vi "Autolocate Fiducials.vi"(6 "FD Index":i32, 8 "error in":errorcluster, 9 "Past Fiducials":dbl[](array[numeric]), 10 "Component":T1, 11 "Gantry In":refnum<k24>) -> (0 "error out":errorcluster, 1 "Wrong Orientation?":bool, 2 "Component Out":T1, 3 "Gantry Out":refnum<k24>)   [LabVIEW 2021, in "Component Tray.lvclass"]
uses:
  Component Tray.lvclass
  C:/Program Files (x86)/Aerotech/A3200/LabVIEW/2010/Bin/Aerotech.A3200.dll
  Program Files (x86)/Aerotech/A3200/LabVIEW/2010/Bin/Aerotech.A3200.dll
  Find Component.ctl
  Controller/Camera/Machine Vision.ctl
  Controller/Motion/A3200/A3200.lvclass
  Controller/Motion/Motion.lvclass
  Controller/Camera/Camera.lvclass
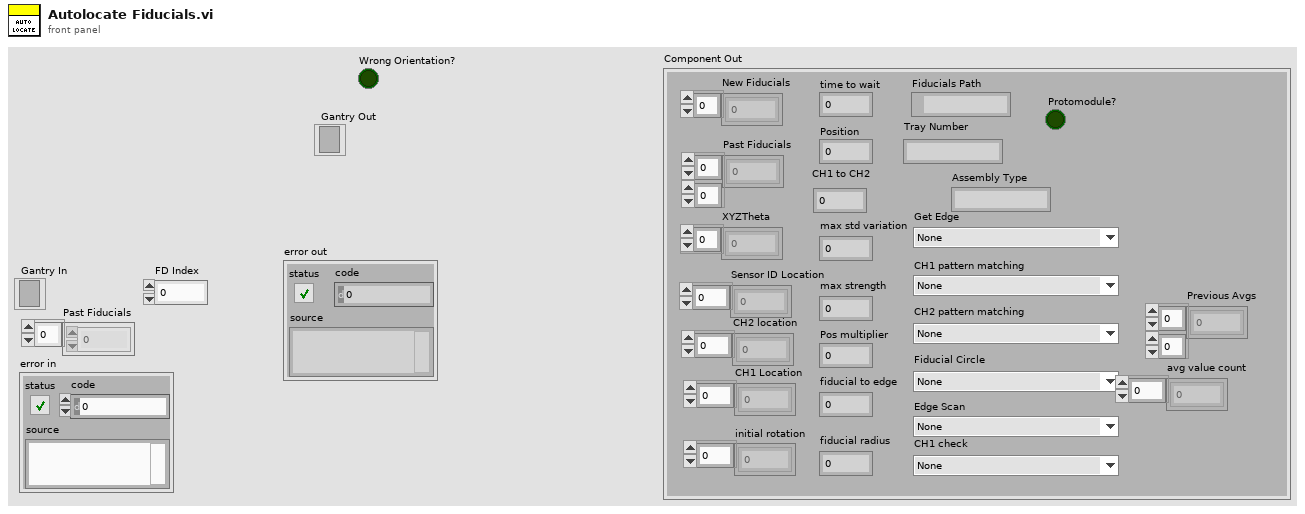
[diagram p1: front panel]
types:
  T1 = typedef "Component Tray.lvclass/Find Component.ctl" = cluster{"New Fiducials":dbl[], "Past Fiducials":dbl[][], "XYZTheta":dbl[], "Fiducials Path":path, "Position":i32, "CH1 Location":dbl[], "Sensor ID Location":dbl[], "initial rotation":dbl[], "CH2 location":dbl[], "max std variation":dbl, "max strength":dbl, "CH2 pattern matching":T2, "Fiducial Circle":T2, "Get Edge":T2, "Pos multiplier":dbl, "time to wait":u32, "fiducial to edge":dbl, "Protomodule?":bool, "Assembly Type":string, "CH1 to CH2":dbl, "Tray Number":string, "fiducial radius":dbl, "4 fiducials?":bool, "CH1 check":T2, "Edge Scan":T2, "CH1 pattern matching":T2, "Sensor Thickness":dbl, "Previous Avgs":dbl[][], "avg value count":dbl[]}
  T2 = typedef "Camera.lvclass/Machine Vision.ctl" = enum16{"None", "Assembly Tray Circle", "Assembly Tray Fiducial", "Partial Hexaboard", "sensor edge init", "HB edge init", "sensor edge pos1", "sensor edge pos2", "HB edge pos1", "HB edge pos2", "Sensor CH1-2", "HB CH1", "HB CH2", "V3 Sensor Circle", "Hexaboard Circle", "sensor CH1 check", "HB CH1 check ", "sensor ID"}
  T3 = enum16{"None", "Assembly Tray Circle", "Assembly Tray Fiducial", "Partial Hexaboard", "sensor edge init", "HB edge init", "sensor edge pos1", "sensor edge pos2", "HB edge pos1", "HB edge pos2", "Sensor CH1-2", "HB CH1", "HB CH2", "V3 Sensor Circle", "Hexaboard Circle", "sensor CH1 check", "HB CH1 check "}
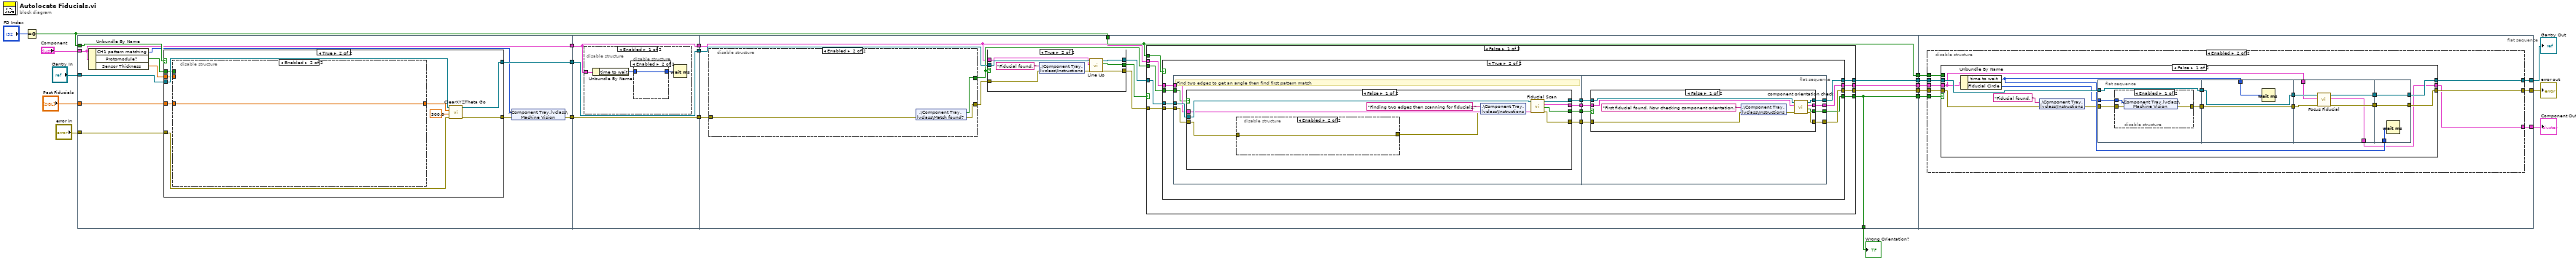
[diagram p0: block diagram]
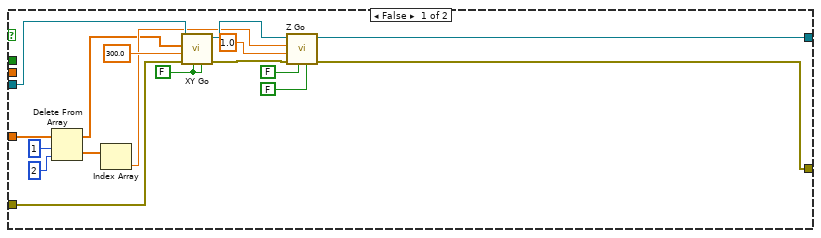
[diagram p2: hidden frame]
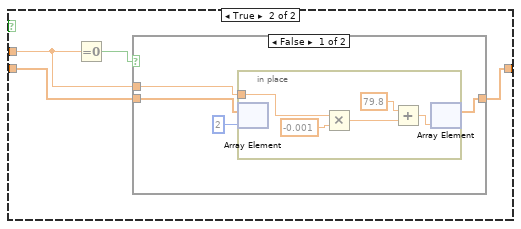
[diagram p4: hidden frame]
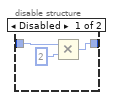
[diagram p6: hidden frame]
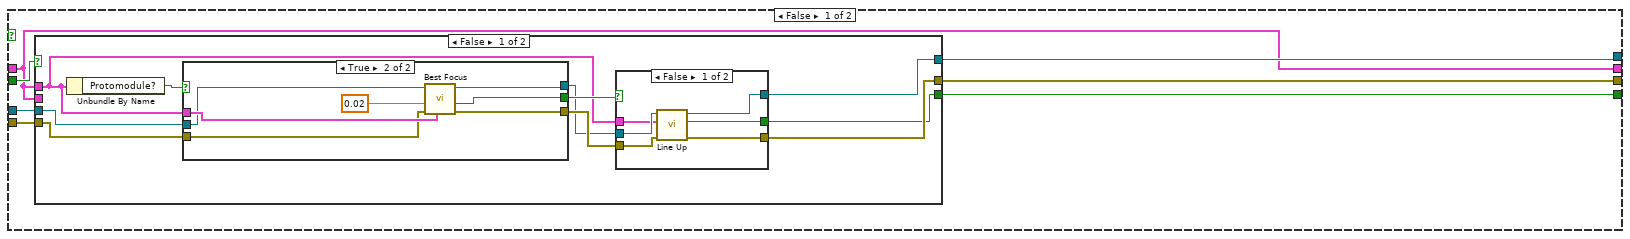
[diagram p8: hidden frame]
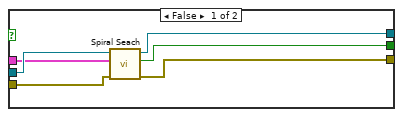
[diagram p9: hidden frame]
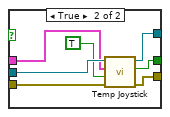
[diagram p10: hidden frame]
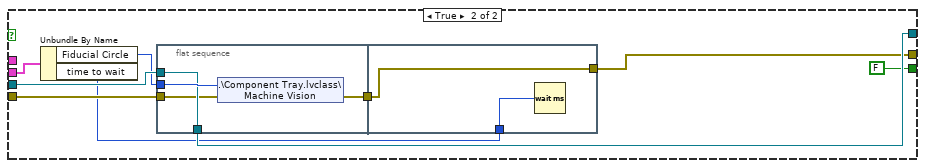
[diagram p11: hidden frame]
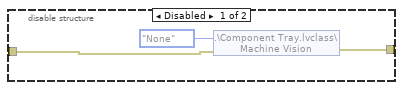
[diagram p12: hidden frame]
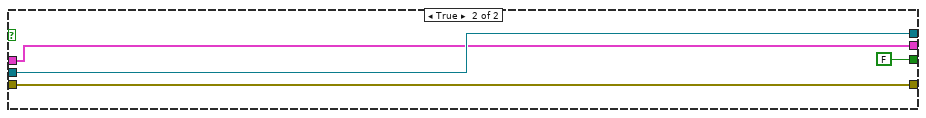
[diagram p13: hidden frame]
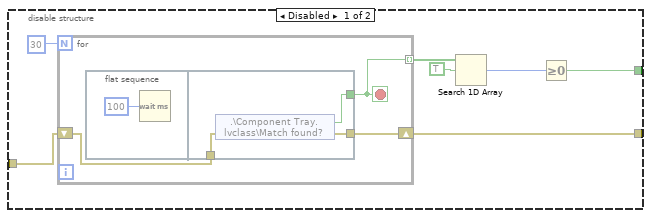
[diagram p16: hidden frame]
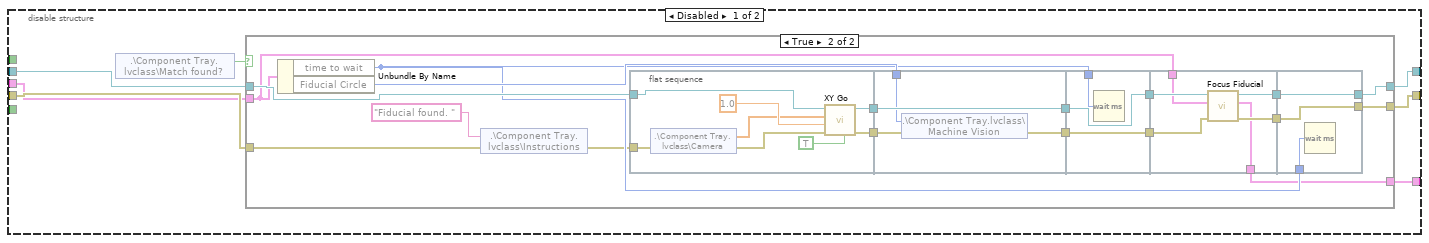
[diagram p18: hidden frame]
diagram:
  n1 = Equal To 0?(x="FD Index") -> (x = 0?=w17:bool)
  n2 = flat-sequence {
    tunnel: w17 -> [w32]
    tunnel: "Gantry In" -> [w31]
    tunnel: "Past Fiducials" -> [w30]
    tunnel: "error in" -> [w24]
    tunnel: [w29] -> w10
    tunnel: "Component" -> [w28]
    tunnel: [w28] -> w11
    tunnel: [w22] -> w9
    tunnel: w11 -> [w81]
    tunnel: [w81] -> w6
    tunnel: [w80] -> w5
    tunnel: w10 -> [w79]
    tunnel: [w79] -> w4
    tunnel: w9 -> [w80]
    tunnel: w17 -> [w97]
    tunnel: [w101] -> w16
    tunnel: [w99] -> w15
    tunnel: [w100] -> w13
    tunnel: [w98] -> w12
    tunnel: [w98] -> w8
    tunnel: [w97] -> w7
    tunnel: w4 -> [w93]
    tunnel: w5 -> [w96]
    tunnel: w6 -> [w90]
    tunnel: [w267] -> w1
    tunnel: [w266] -> w3
    tunnel: w16 -> [w265]
    tunnel: w15 -> [w263]
    tunnel: [w262] -> w2
    tunnel: w13 -> [w264]
    tunnel: w8 -> [w261]
    tunnel: w7 -> [w260]
    frame #0 {
      n3 = Unbundle By Name(w28) -> ("CH1 pattern matching"=w27:T2, "Protomodule?"=w26:bool, "Sensor Thickness"=w25:dbl)
      n4 = case shown="True" w32 {
        tunnel: w30 -> [w45 w54]
        tunnel: w31 -> [w49 w58]
        tunnel: [w43 w57] -> w29
        tunnel: w24 -> [w47 w56]
        tunnel: w26 -> [_ w50]
        tunnel: [w42 w55] -> w23
        tunnel: w25 -> [_ w53]
        frame False {
          w48 = FALSE ("Increment?")
          n5 = Delete From Array(array=w45, length=1, index=2) -> (deleted portion=w35:dbl[], array with subset deleted=w33:dbl[])
          n6 = Index Array(array=w35) -> (element=w34:dbl)  [unwired: 1 in]
          n7 = call "XY Go.vi"("Increment?"=w48, "return immediately"=w48, "error in (no error)"=w47, "Speed"=300.0, "XY In"=w33, "Gantry In"=w49) -> ("error out"=w41:errorcluster, "Gantry Out"=w44:refnum<k24>)  [unwired: 3 in, 1 out]
          n8 = call "Z Go.vi"("Increment"=FALSE, "Return Immediately"=FALSE, "error in (no error)"=w41, "Speed In"=1.0, "Position In"=w34, "Gantry In"=w44) -> ("error out"=w42:errorcluster, "Gantry Out"=w43:refnum<k24>)  [unwired: 2 in, 2 out]
        }
        frame True {
          n9 = disable-structure shown="Enabled" {
            disable-tunnel: w54 -> [w62 w78]
            disable-tunnel: w53 -> [w61 _]
            disable-tunnel: [w60 w78] -> w52
            disable-tunnel: w50 -> [w59 _]
            frame Disabled {
              n10 = case shown="False" w59 {
                tunnel: w62 -> [w63 w66]
                tunnel: w61 -> [_ w65]
                tunnel: [w63 w64] -> w60
                frame False {
                }
                frame True {
                  n11 = Equal To 0?(x=w65) -> (x = 0?=w67:bool)
                  n12 = case shown="False" w67 {
                    tunnel: w66 -> [w71 w77]
                    tunnel: w65 -> [w70 _]
                    tunnel: [w69 w77] -> w64
                    frame False {
                      n13 = in-place {
                        in-place-border: w70 -> [w75]
                        n14 = in-place-array #1(w71, 2) -> ()  [unwired: 1 out]
                        n15 = Multiply(x=w75, y=-0.001) -> (x*y=w73:dbl)
                        n16 = Add(x=79.8, y=w73) -> (x+y=w72:dbl)
                        n17 = in-place-array #1(w72) -> (w69:dbl[])  [unwired: 1 out]
                      }
                    }
                    frame True {
                    }
                  }
                }
              }
            }
            frame Enabled {
            }
          }
          n18 = call "ClearXYZTheta Go.vi"("error in (no error)"=w56, "Speed"=300.0, "XYZTheta In"=w52, "Gantry In"=w58) -> ("error out"=w55:errorcluster, "Gantry Out"=w57:refnum<k24>)  [unwired: 5 in, 1 out]
        }
      }
      n19 = shared-variable ".\\Component Tray.lvclass\\Machine Vision"(w27, error in=w23) -> (error out=w22:errorcluster)
    }
    frame #1 {
      n20 = disable-structure shown="Enabled" {
        disable-tunnel: w81 -> [w84 _]
        frame Enabled {
          n21 = Unbundle By Name(w84) -> ("time to wait"=w83:u32)
          n22 = disable-structure shown="Enabled" {
            disable-tunnel: w83 -> [w87 w88]
            disable-tunnel: [w85 w88] -> w82
            frame Disabled {
              n23 = Multiply(x=w87, y=u32 2) -> (x*y=w85:u32)
            }
            frame Enabled {
            }
          }
          n24 = Wait (ms)(milliseconds to wait=w82) -> ()  [unwired: 1 out]
        }
        frame Disabled {
        }
      }
    }
    frame #2 {
      n25 = disable-structure shown="Enabled" {
        disable-tunnel: w96 -> [w238 w247]
        disable-tunnel: [w236 w248] -> w95
        disable-tunnel: [w232 w246] -> w91
        frame Disabled {
          n26 = for {
            N: 30 -> [_]
            tunnel: [w240] -> w235 mode=indexing
            shift-right: [w239] -> w236
            shift-left: w238 -> [w241]
            stop <- w240 stop-if-true
            n27 = flat-sequence {
              tunnel: w241 -> [w245]
              tunnel: [w244] -> w240
              tunnel: [w243] -> w239
              frame #0 {
                n28 = Wait (ms)(milliseconds to wait=u32 100) -> ()  [unwired: 1 out]
              }
              frame #1 {
                n29 = shared-variable ".\\Component Tray.lvclass\\Match found?"(error in=w245) -> (w244:bool, error out=w243:errorcluster)
              }
            }
          }
          n30 = Search 1D Array(1D array=w235, element=TRUE) -> (index of element=w233:i32)  [unwired: 1 in]
          n31 = Greater Or Equal To 0?(x=w233) -> (x >= 0?=w232:bool)
        }
        frame Enabled {
          n32 = shared-variable ".\\Component Tray.lvclass\\Match found?"(error in=w247) -> (w246:bool, error out=w248:errorcluster)
        }
      }
      n33 = case shown="True" w91 {
        selector: w91 -> [w249 _]
        tunnel: w95 -> [w251 w258]
        tunnel: [w251 w254] -> w94
        tunnel: w93 -> [w250 w257]
        tunnel: [w250 w256] -> w92
        tunnel: w90 -> [_ w253]
        tunnel: [w249 w252] -> w89
        frame False {
        }
        frame True {
          n34 = shared-variable ".\\Component Tray.lvclass\\Instructions"("Fiducial found. " ("Instructions"), error in=w258) -> (error out=w255:errorcluster)
          n35 = call "Line Up.vi"("error IO"=w255, "Component"=w253, "Gantry In"=w257) -> ("error out"=w254:errorcluster, "Error?"=w252:bool, "Gantry Out"=w256:refnum<k24>)  [unwired: 6 in]
        }
      }
      n36 = case shown="False" w89 {
        selector: w89 -> [_ w229]
        tunnel: [w110 w231] -> w101
        tunnel: [w109 w230] -> w100
        tunnel: [w108 w228] -> w99
        tunnel: [w107 w229] -> w98
        tunnel: w97 -> [w106 _]
        tunnel: w94 -> [w105 w230]
        tunnel: w92 -> [w104 w231]
        tunnel: w91 -> [w103 _]
        tunnel: w90 -> [w102 w228]
        frame False {
          n37 = case shown="True" w106 {
            tunnel: w104 -> [w117 w180]
            tunnel: [w116 w179] -> w110
            tunnel: [w115 w178] -> w109
            tunnel: w102 -> [w111 w177]
            tunnel: [w111 w176] -> w108
            tunnel: [w112 w172] -> w107
            tunnel: w103 -> [w113 w170]
            tunnel: w105 -> [w114 w169]
            frame False {
              n38 = case shown="False" w113 {
                tunnel: w114 -> [w124 w162]
                tunnel: w117 -> [w123 w161]
                tunnel: w111 -> [_ w159]
                tunnel: [w127 w160] -> w116
                tunnel: [w126 w157] -> w115
                tunnel: [w118 FALSE ("Wrong Orientation?")] -> w112
                tunnel: w111 -> [w119 _]
                frame False {
                  n39 = Unbundle By Name(w119) -> ("Protomodule?"=w125:bool)
                  n40 = case shown="True" w125 {
                    tunnel: w119 -> [w128 w140]
                    tunnel: w124 -> [w129 w139]
                    tunnel: w123 -> [w133 w138]
                    tunnel: [w130 w137] -> w122
                    tunnel: [w131 w136] -> w121
                    tunnel: [w132 w135] -> w120
                    frame False {
                      n41 = call "Spiral Seach.vi"("error in (no error)"=w129, "Component"=w128, "Gantry In"=w133) -> ("error out"=w130:errorcluster, "Error?"=w131:bool, "Gantry Out"=w132:refnum<k24>)  [unwired: 6 in]
                    }
                    frame True {
                      n42 = call "Best Focus.vi"("Component"=w140, "error in (no error)"=w139, "Inc by"=0.02 ("Start"), "Gantry In"=w138) -> ("error out"=w137:errorcluster, "Error?"=w136:bool, "Gantry Out"=w135:refnum<k24>)  [unwired: 4 in, 1 out]
                    }
                  }
                  n43 = case shown="False" w121 {
                    tunnel: w120 -> [w146 w153]
                    tunnel: [w145 w152] -> w127
                    tunnel: [w144 w148] -> w126
                    tunnel: w122 -> [w143 w149]
                    tunnel: w119 -> [w142 w151]
                    tunnel: [w141 w147] -> w118
                    frame False {
                      n44 = call "Line Up.vi"("error IO"=w143, "Component"=w142, "Gantry In"=w146) -> ("error out"=w144:errorcluster, "Error?"=w141:bool, "Gantry Out"=w145:refnum<k24>)  [unwired: 6 in]
                    }
                    frame True {
                      n45 = call "Temp Joystick.vi"("error in (no error)"=w149, "Fiducial?"=TRUE, "Component"=w151, "Gantry In"=w153) -> ("error out"=w148:errorcluster, "Error?"=w147:bool, "Gantry Out"=w152:refnum<k24>)  [unwired: 5 in]
                    }
                  }
                }
                frame True {
                  n46 = Unbundle By Name(w159) -> ("Fiducial Circle"=w158:T2, "time to wait"=w155:u32)
                  n47 = flat-sequence {
                    tunnel: w158 -> [w166]
                    tunnel: [w165] -> w156
                    tunnel: w162 -> [w163]
                    tunnel: [w164] -> w160
                    tunnel: w161 -> [w164]
                    tunnel: [w168] -> w157
                    tunnel: w156 -> [w168]
                    tunnel: w155 -> [w167]
                    frame #0 {
                      n48 = shared-variable ".\\Component Tray.lvclass\\Machine Vision"(w166, error in=w163) -> (error out=w165:errorcluster)
                    }
                    frame #1 {
                      n49 = Wait (ms)(milliseconds to wait=w167) -> ()  [unwired: 1 out]
                    }
                  }
                }
              }
            }
            frame True {
              n50 = flat-sequence {
                tunnel: w180 -> [w188]
                tunnel: w177 -> [w185]
                tunnel: [w187] -> w175
                tunnel: [w186] -> w174
                tunnel: [w184] -> w173
                tunnel: [w183] -> w171
                tunnel: w170 -> [w182]
                tunnel: w169 -> [w181]
                tunnel: [w211] -> w176
                tunnel: [w213] -> w178
                tunnel: [w214] -> w179
                tunnel: [w212] -> w172
                tunnel: w173 -> [w208]
                tunnel: w174 -> [w209]
                tunnel: w175 -> [w210]
                tunnel: w171 -> [w207]
                frame #0 {
                  # "Find two edges to get an angle then find first pattern match"
                  n51 = case shown="False" w182 {
                    tunnel: w188 -> [w198 w206]
                    tunnel: [w197 w206] -> w187
                    tunnel: w181 -> [w191 w205]
                    tunnel: [w196 w205] -> w186
                    tunnel: w185 -> [w195 w204]
                    tunnel: [w194 w204] -> w184
                    tunnel: [w193 FALSE] -> w183
                    frame False {
                      n52 = disable-structure shown="Enabled" {
                        disable-tunnel: w191 -> [w200 w202]
                        disable-tunnel: [w199 w202] -> w190
                        frame Disabled {
                          n53 = shared-variable ".\\Component Tray.lvclass\\Machine Vision"(T3."None" ("Machine Vision"), error in=w200) -> (error out=w199:errorcluster)
                        }
                        frame Enabled {
                        }
                      }
                      n54 = shared-variable ".\\Component Tray.lvclass\\Instructions"("Finding two edges then scanning for fiducials." ("Instructions"), error in=w190) -> (error out=w189:errorcluster)
                      n55 = call "Fiducial Scan.vi"("error in"=w189, "input cluster"=w195, "Gantry In"=w198) -> ("error out"=w196:errorcluster, "Not Found?"=w193:bool, "output cluster"=w194:T1, "Gantry Out"=w197:refnum<k24>)  [unwired: 5 in]
                    }
                    frame True {
                    }
                  }
                }
                frame #1 {
                  n56 = case shown="False" w207 {
                    selector: w207 -> [_ w224]
                    tunnel: [w223 w227] -> w214
                    tunnel: [w222 w225] -> w213
                    tunnel: [w221 w224] -> w212
                    tunnel: [w220 w226] -> w211
                    tunnel: w210 -> [w218 w227]
                    tunnel: w209 -> [w216 w225]
                    tunnel: w208 -> [w219 w226]
                    frame False {
                      n57 = shared-variable ".\\Component Tray.lvclass\\Instructions"("First fiducial found. Now checking component orientation." ("Instructions"), error in=w216) -> (error out=w215:errorcluster)
                      n58 = call "component orientation check.vi"("error in"=w215, "input cluster"=w219, "Gantry In"=w218) -> ("error out"=w222:errorcluster, "Wrong Orientation?"=w221:bool, "output cluster"=w220:T1, "Gantry Out"=w223:refnum<k24>)  [unwired: 5 in]
                    }
                    frame True {
                    }
                  }
                }
              }
            }
          }
        }
        frame True {
        }
      }
    }
    frame #3 {
      n59 = disable-structure shown="Enabled" {
        disable-tunnel: [w274 w324] -> w267
        disable-tunnel: [w273 w323] -> w266
        disable-tunnel: w265 -> [w272 w327]
        disable-tunnel: w264 -> [w271 w326]
        disable-tunnel: w263 -> [w270 w325]
        disable-tunnel: [w269 w322] -> w262
        disable-tunnel: w261 -> [_ w321]
        disable-tunnel: w260 -> [_ w320]
        frame Disabled {
          n60 = shared-variable ".\\Component Tray.lvclass\\Match found?"() -> (w268:bool)  [unwired: 1 in, 1 out]
          n61 = case shown="True" w268 {
            tunnel: w272 -> [w277 w295]
            tunnel: [w277 w294] -> w274
            tunnel: w271 -> [w275 w279]
            tunnel: w270 -> [w276 w290]
            tunnel: [w275 w291] -> w273
            tunnel: [w276 w281] -> w269
            frame False {
            }
            frame True {
              n62 = Unbundle By Name(w290) -> ("time to wait"=w282:u32, "Fiducial Circle"=w287:T2)
              n63 = shared-variable ".\\Component Tray.lvclass\\Instructions"("Fiducial found. " ("Instructions"), error in=w279) -> (error out=w278:errorcluster)
              n64 = flat-sequence {
                tunnel: w295 -> [w303]
                tunnel: w278 -> [w297]
                tunnel: [w302] -> w293
                tunnel: [w299] -> w292
                tunnel: w293 -> [w307]
                tunnel: [w307] -> w286
                tunnel: w292 -> [w305]
                tunnel: [w304] -> w284
                tunnel: w287 -> [w306]
                tunnel: w286 -> [w310]
                tunnel: [w310] -> w285
                tunnel: w284 -> [w309]
                tunnel: [w309] -> w283
                tunnel: w282 -> [w308]
                tunnel: w285 -> [w314]
                tunnel: w283 -> [w313]
                tunnel: w290 -> [w312]
                tunnel: [w316] -> w289
                tunnel: [w315] -> w288
                tunnel: [w311] -> w281
                tunnel: [w318] -> w291
                tunnel: [w319] -> w294
                tunnel: w289 -> [w319]
                tunnel: w288 -> [w318]
                tunnel: w282 -> [w317]
                frame #0 {
                  n65 = shared-variable ".\\Component Tray.lvclass\\Camera"(error in=w297) -> (w298:dbl[], error out=w296:errorcluster)
                  n66 = call "XY Go.vi"("Increment?"=TRUE, "error in (no error)"=w296, "Speed"=1.0, "XY In"=w298, "Gantry In"=w303) -> ("error out"=w299:errorcluster, "Gantry Out"=w302:refnum<k24>)  [unwired: 4 in, 1 out]
                }
                frame #1 {
                  n67 = shared-variable ".\\Component Tray.lvclass\\Machine Vision"(w306, error in=w305) -> (error out=w304:errorcluster)
                }
                frame #2 {
                  n68 = Wait (ms)(milliseconds to wait=w308) -> ()  [unwired: 1 out]
                }
                frame #3 {
                  n69 = call "Focus Fiducial.vi"("error in"=w313, "Component In"=w312, "Gantry In"=w314) -> ("error out"=w315:errorcluster, "Component Out"=w311:T1, "Gantry Out"=w316:refnum<k24>)  [unwired: 6 in]
                }
                frame #4 {
                  n70 = Wait (ms)(milliseconds to wait=w317) -> ()  [unwired: 1 out]
                }
              }
            }
          }
        }
        frame Enabled {
          n71 = case shown="False" w321 {
            tunnel: w327 -> [w343 w366]
            tunnel: [w342 w366] -> w324
            tunnel: w326 -> [w329 w364]
            tunnel: w325 -> [w340 w365]
            tunnel: [w341 w364] -> w323
            tunnel: [w332 w365] -> w322
            tunnel: w320 -> [_ _]
            frame False {
              n72 = Unbundle By Name(w340) -> ("time to wait"=w333:u32, "Fiducial Circle"=w328:T2)
              n73 = shared-variable ".\\Component Tray.lvclass\\Instructions"("Fiducial found. " ("Instructions"), error in=w329) -> (error out=w330:errorcluster)
              n74 = flat-sequence {
                tunnel: [w344] -> w337
                tunnel: [w346] -> w335
                tunnel: w328 -> [w347]
                tunnel: w330 -> [w345]
                tunnel: w343 -> [w344]
                tunnel: w337 -> [w354]
                tunnel: [w354] -> w336
                tunnel: w335 -> [w353]
                tunnel: [w353] -> w334
                tunnel: w333 -> [w352]
                tunnel: w336 -> [w358]
                tunnel: w334 -> [w357]
                tunnel: w340 -> [w356]
                tunnel: [w360] -> w339
                tunnel: [w359] -> w338
                tunnel: [w355] -> w332
                tunnel: [w362] -> w341
                tunnel: [w363] -> w342
                tunnel: w339 -> [w363]
                tunnel: w338 -> [w362]
                tunnel: w333 -> [w361]
                frame #0 {
                  n75 = disable-structure shown="Enabled" {
                    disable-tunnel: w347 -> [w350 _]
                    disable-tunnel: w345 -> [w349 w351]
                    disable-tunnel: [w348 w351] -> w346
                    frame Enabled {
                      n76 = shared-variable ".\\Component Tray.lvclass\\Machine Vision"(w350, error in=w349) -> (error out=w348:errorcluster)
                    }
                    frame Disabled {
                    }
                  }
                }
                frame #1 {
                  n77 = Wait (ms)(milliseconds to wait=w352) -> ()  [unwired: 1 out]
                }
                frame #2 {
                  n78 = call "Focus Fiducial.vi"("error in"=w357, "Component In"=w356, "Gantry In"=w358) -> ("error out"=w359:errorcluster, "Component Out"=w355:T1, "Gantry Out"=w360:refnum<k24>)  [unwired: 6 in]
                }
                frame #3 {
                  n79 = Wait (ms)(milliseconds to wait=w361) -> ()  [unwired: 1 out]
                }
              }
            }
            frame True {
            }
          }
        }
      }
    }
  }
  "Gantry Out" <- w1
  "error out" <- w3
  "Component Out" <- w2
  "Wrong Orientation?" <- w12
